vi "Benchmark FIFO delay.vi"() -> ()   [LabVIEW 2011]
uses:
  <vilib>/Platform/TimedLoop/XDataNode/timing_clust.ctl
  <vilib>/Platform/TimedLoop/XDataNode/nitl_modes.ctl
  <vilib>/Platform/TimedLoop/XDataNode/wakeup.ctl
  <vilib>/rvi/DataTransferAndStorage/Container/Common/niFpgaContainerExecOnDevCompGetState.vi
  <vilib>/rvi/FIFO/Fifo_Resource/nirvififoEmulationSetSize.vi
  <vilib>/rvi/DataTransferAndStorage/Container/Common/niFpgaContainerGetUniqueNameForEmu.vi
  <vilib>/rvi/interface/RandomDataEmulation/nirviRandomDataFPGAFIFO.vi
  <vilib>/rvi/interface/RandomDataEmulation/niFpgaRandomDataHandleErrors.vi
  <vilib>/rvi/eio/common/nirviEmuReportErrorAndStop.vi
  <vilib>/Platform/TimedLoop/XDataNode/XDataNode.xnode
  <vilib>/rvi/DataTransferAndStorage/Container/XNode/niFpgaContainer.xnode
  <vilib>/rvi/FIFO/Fifo_Resource/niFpgaFifoEmulationRefIn.vi
  <vilib>/rvi/FXPMathLib/basic elements/FxpDiscreteDelay/XNode/nifxpmath_DiscreteDelay.xnode
  <vilib>/Platform/TimedLoop/XDataNode/XDNodeRunTimeDep.lvlib
panel:
  out "Out":i16[](array[numeric])
  out "Write[N-7]":bool
  in  "Input":i16[](array[numeric])=[0, 0, 0, 0, 0, 0, 0, 0]
  out "Out1":i16[](array[numeric])
  out "Write[N-6]":bool
  out "Write[N-5]":bool
  out "Write[N-4]":bool
  out "Write[N-3]":bool
  out "Write[N-2]":bool
  out "Write[N-1]":bool
  out "Write[N]":bool
  in  "Write":bool
  # "200M -> N-5"
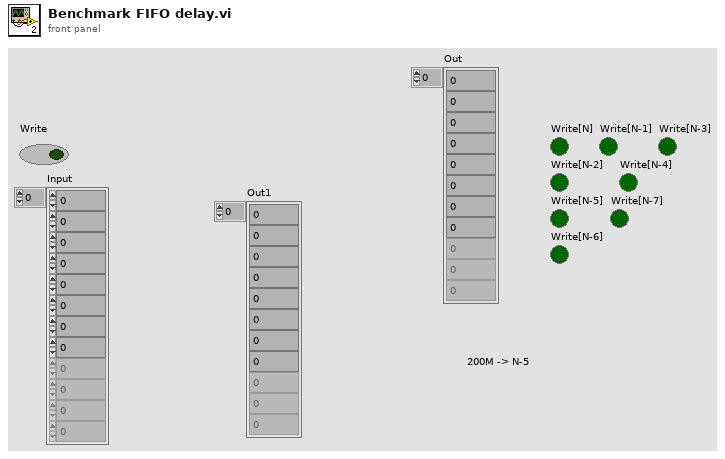
[diagram p1: front panel]
types:
  T1 = typedef "XDNodeRunTimeDep.lvlib/timing_clust.ctl" = cluster{"Expected End [f-1]":u64, "Actual End [f-1]":u64, "Finished Late? [f-1]":bool, "Expected End [i-1]":u64, "Actual End [i-1]":u64, "Finished Late? [i-1]":bool, "Expected Start [i]":u64, "Actual Start [i]":u64, "Expected Start [f]":u64, "Actual Start [f]":u64, "Source Name":string, "Structure Name":string, "Period":i64, "Deadline":i64, "Offset":i64, "Start":i64, "Priority":i32, "Timeout":i32, "Mode":T2, "Wakeup Reason":T3, "Error":errorcluster, "Source Type":string, "Secondary Source Type":string, "Global End Time":u64, "Global Start Time":u64, "Frame Duration":u64, "Iteration Duration":u64, "Assigned CPU":i32, "I/O Scan Engine Mode":u32}
  T2 = typedef "XDNodeRunTimeDep.lvlib/nitl_modes.ctl" = enum32{"No Change", "Process missed periods, maintain original phase", "Discard missed periods, maintain original phase", "Process missed periods, ignore original phase", "Discard missed periods, ignore original phase"}
  T3 = typedef "XDNodeRunTimeDep.lvlib/wakeup.ctl" = enum32{"Normal", "Aborted", "Asynchronous wakeup", "Timing source error", "Timed loop error", "Timeout"}
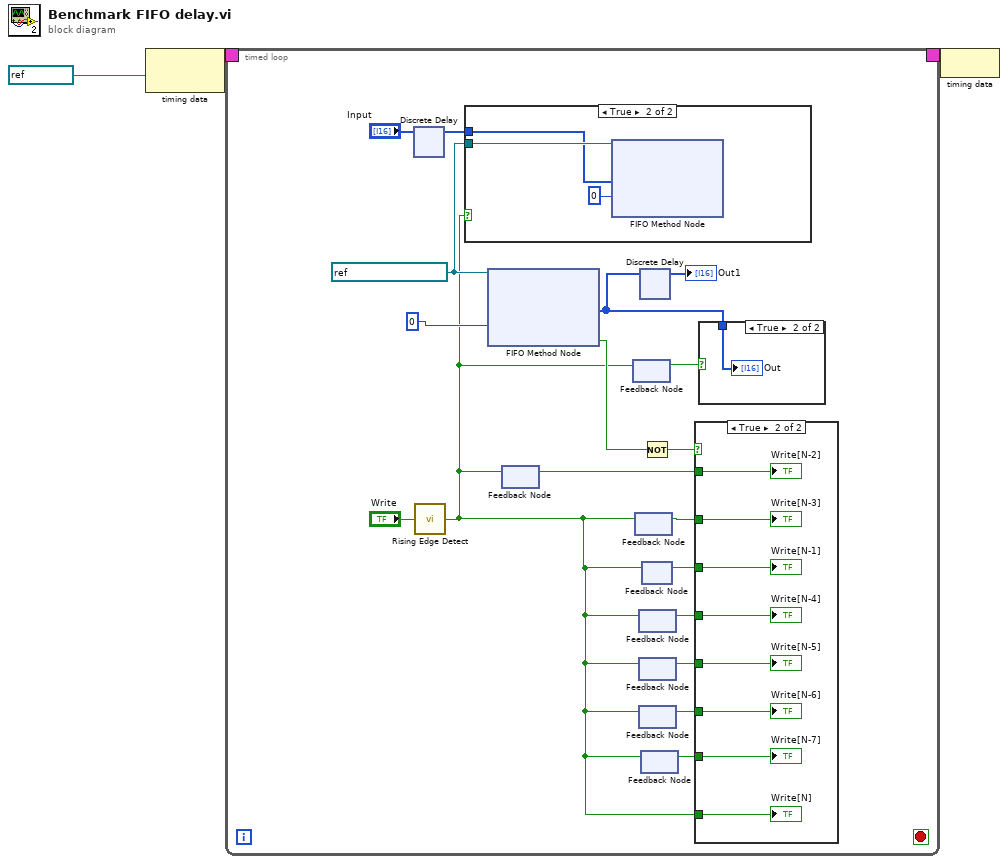
[diagram p0: block diagram]
diagram:
  n1 = node-c288(refnum<k21> "80MHz" ("Source Name")) -> (w3:T1)
  n2 = timed-loop {
    timing: w3 -> [_]
    timing-out: [_] -> w2
    stop <- _ stop-if-true
    w21 = refnum<k21> "HistoryFIFOU128" ("FIFO Out")
    n3 = xnode "Discrete Delay"("D"="Input") -> ("Q"=w8:i16[])
    n4 = call <userlib>:"Rising Edge Detect.vi"("signal"="Write") -> ("edge detected"=w5:bool)  [unwired: 14 in]
    n5 = case shown="True" w5 {
      tunnel: w21 -> [_ w33]
      tunnel: w8 -> [_ w31]
      frame False {
      }
      frame True {
        n6 = xnode ("FIFO Method Node")("Element"=w31, "Timeout"=0, "FIFO In"=w33) -> ()  [unwired: 2 out]
      }
    }
    n7 = xnode ("FIFO Method Node")("Timeout"=0, "FIFO In"=w21) -> ("Element"=w4:i16[], "Timed Out?"=w19:bool)  [unwired: 1 out]
    n8 = feedback #1() -> (w13:bool)  [unwired: 1 in]
    n9 = feedback-in #1(w5) -> ()
    n10 = feedback #2() -> (w6:bool)  [unwired: 1 in]
    n11 = feedback-in #2(w5) -> ()
    n12 = feedback #3() -> (w14:bool)  [unwired: 1 in]
    n13 = feedback-in #3(w5) -> ()
    n14 = feedback #4() -> (w15:bool)  [unwired: 1 in]
    n15 = feedback-in #4(w5) -> ()
    n16 = feedback #5() -> (w12:bool)  [unwired: 1 in]
    n17 = feedback-in #5(w5) -> ()
    n18 = feedback #6() -> (w11:bool)  [unwired: 1 in]
    n19 = feedback-in #6(w5) -> ()
    n20 = xnode "Discrete Delay"("D"=w4) -> ("Q"=→"Out1":i16[])
    n21 = feedback #7() -> (w7:bool)  [unwired: 1 in]
    n22 = feedback-in #7(w5) -> ()
    n23 = Not(x=w19) -> (.not. x?=w17:bool)
    n24 = feedback #8() -> (w16:bool)  [unwired: 1 in]
    n25 = feedback-in #8(w5) -> ()
    n26 = case shown="True" w17 {
      tunnel: w5 -> [_ w30]
      tunnel: w16 -> [_ w29]
      tunnel: w15 -> [_ w26]
      tunnel: w14 -> [_ w27]
      tunnel: w13 -> [_ w28]
      tunnel: w12 -> [_ w25]
      tunnel: w11 -> [_ w24]
      tunnel: w7 -> [_ w23]
      frame False {
      }
      frame True {
        "Write[N]" <- w30
        "Write[N-1]" <- w29
        "Write[N-2]" <- w28
        "Write[N-3]" <- w27
        "Write[N-4]" <- w26
        "Write[N-5]" <- w25
        "Write[N-6]" <- w24
        "Write[N-7]" <- w23
      }
    }
    n27 = case shown="True" w6 {
      tunnel: w4 -> [_ w22]
      frame False {
      }
      frame True {
        "Out" <- w22
      }
    }
  }
  n28 = node-c288(w2) -> ()
